vi "Generate Signal.vi"(8 "error in (no error)":errorcluster, 11 "Sampling Rate":dbl=10000000.0 format="%#_13p") -> (0 "error out":errorcluster, 2 "Waveform Out":waveform(cdb))   [LabVIEW 2018]
panel:
  out "Waveform Graph":dbl[](graph)
  out "Sampling Rate [Hz]":dbl
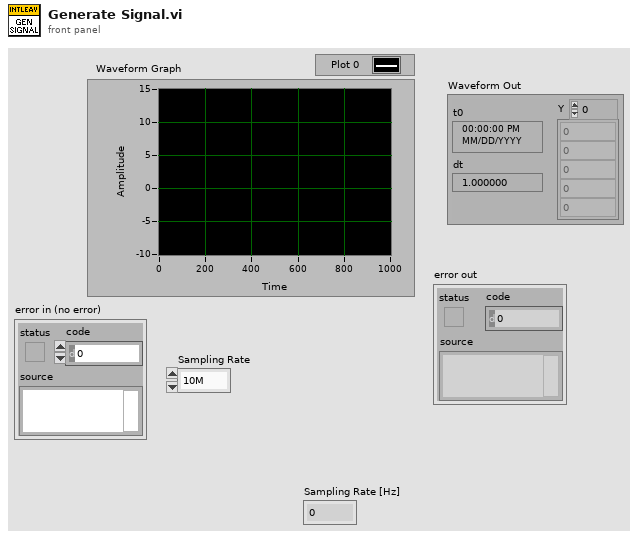
[diagram p1: front panel]
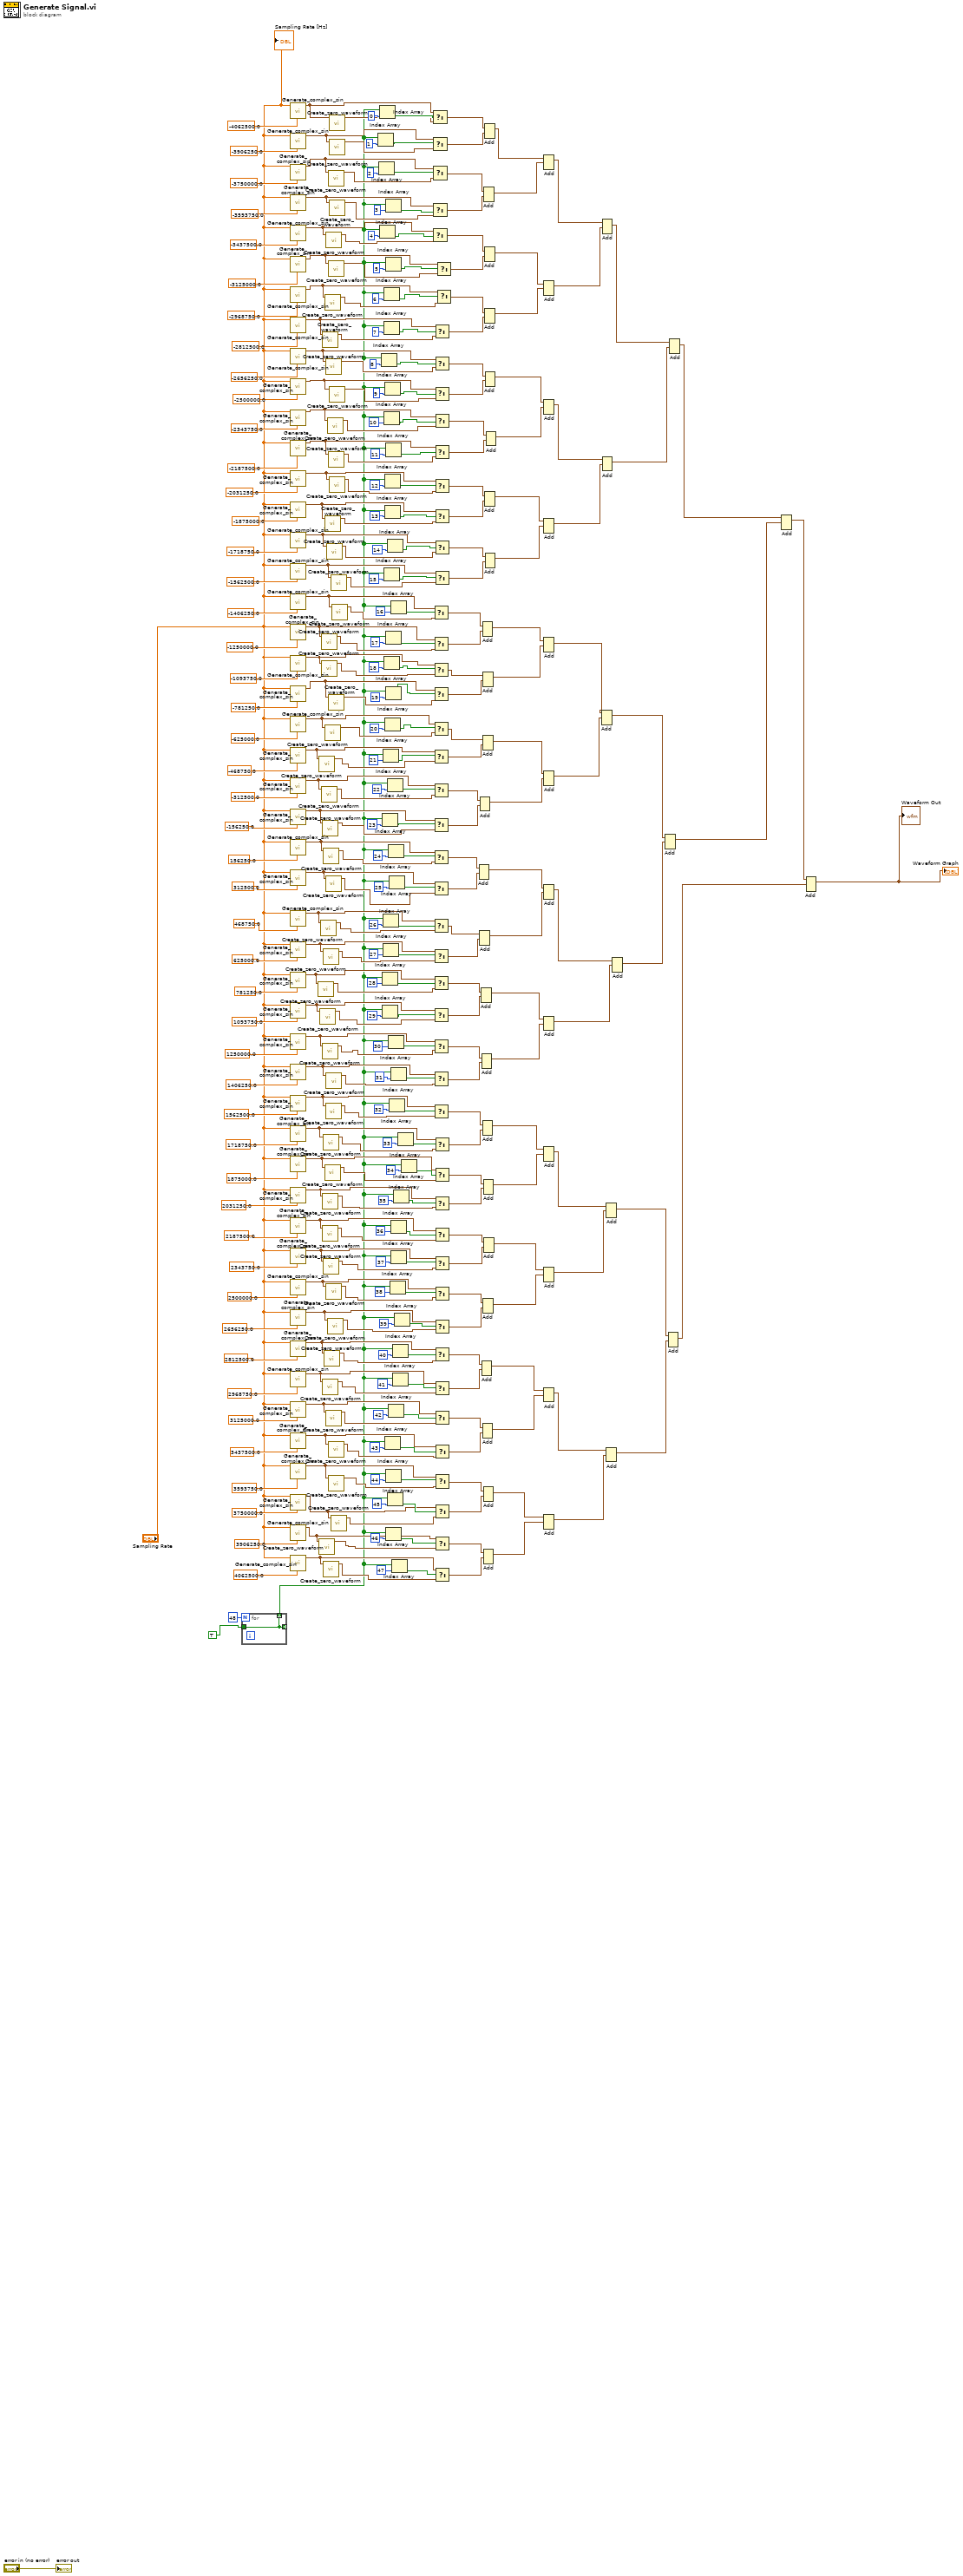
[diagram p0: block diagram]
diagram:
  n1 = for {
    N: 48 -> [_]
    tunnel: TRUE ("Boolean") -> [w341]
    tunnel: [w341] -> _ mode=indexing
    tunnel: [w341] -> w2 mode=indexing
  }
  n2 = call "Generate_complex_sin.vi"("Signal freq"=-4062500.0, "Sampling Rate [Hz]"="Sampling Rate") -> ("Waveform"=w102:waveform(cdb))  [unwired: 9 in]
  n3 = call "Generate_complex_sin.vi"("Signal freq"=-3906250.0, "Sampling Rate [Hz]"="Sampling Rate") -> ("Waveform"=w100:waveform(cdb))  [unwired: 9 in]
  n4 = call "Generate_complex_sin.vi"("Signal freq"=-3750000.0, "Sampling Rate [Hz]"="Sampling Rate") -> ("Waveform"=w97:waveform(cdb))  [unwired: 9 in]
  n5 = call "Generate_complex_sin.vi"("Signal freq"=-3593750.0, "Sampling Rate [Hz]"="Sampling Rate") -> ("Waveform"=w96:waveform(cdb))  [unwired: 9 in]
  n6 = call "Generate_complex_sin.vi"("Signal freq"=-3437500.0, "Sampling Rate [Hz]"="Sampling Rate") -> ("Waveform"=w93:waveform(cdb))  [unwired: 9 in]
  n7 = call "Generate_complex_sin.vi"("Signal freq"=-3125000.0, "Sampling Rate [Hz]"="Sampling Rate") -> ("Waveform"=w92:waveform(cdb))  [unwired: 9 in]
  n8 = call "Generate_complex_sin.vi"("Signal freq"=-2968750.0, "Sampling Rate [Hz]"="Sampling Rate") -> ("Waveform"=w89:waveform(cdb))  [unwired: 9 in]
  n9 = call "Generate_complex_sin.vi"("Signal freq"=-2812500.0, "Sampling Rate [Hz]"="Sampling Rate") -> ("Waveform"=w88:waveform(cdb))  [unwired: 9 in]
  n10 = call "Generate_complex_sin.vi"("Signal freq"=-2656250.0, "Sampling Rate [Hz]"="Sampling Rate") -> ("Waveform"=w86:waveform(cdb))  [unwired: 9 in]
  n11 = call "Generate_complex_sin.vi"("Signal freq"=-2500000.0, "Sampling Rate [Hz]"="Sampling Rate") -> ("Waveform"=w84:waveform(cdb))  [unwired: 9 in]
  n12 = call "Generate_complex_sin.vi"("Signal freq"=-2343750.0, "Sampling Rate [Hz]"="Sampling Rate") -> ("Waveform"=w82:waveform(cdb))  [unwired: 9 in]
  n13 = call "Generate_complex_sin.vi"("Signal freq"=-2187500.0, "Sampling Rate [Hz]"="Sampling Rate") -> ("Waveform"=w80:waveform(cdb))  [unwired: 9 in]
  n14 = call "Generate_complex_sin.vi"("Signal freq"=-2031250.0, "Sampling Rate [Hz]"="Sampling Rate") -> ("Waveform"=w78:waveform(cdb))  [unwired: 9 in]
  n15 = call "Generate_complex_sin.vi"("Signal freq"=-1875000.0, "Sampling Rate [Hz]"="Sampling Rate") -> ("Waveform"=w75:waveform(cdb))  [unwired: 9 in]
  n16 = call "Generate_complex_sin.vi"("Signal freq"=-1718750.0, "Sampling Rate [Hz]"="Sampling Rate") -> ("Waveform"=w74:waveform(cdb))  [unwired: 9 in]
  n17 = call "Generate_complex_sin.vi"("Signal freq"=-1562500.0, "Sampling Rate [Hz]"="Sampling Rate") -> ("Waveform"=w71:waveform(cdb))  [unwired: 9 in]
  n18 = call "Generate_complex_sin.vi"("Signal freq"=-1406250.0, "Sampling Rate [Hz]"="Sampling Rate") -> ("Waveform"=w69:waveform(cdb))  [unwired: 9 in]
  n19 = call "Generate_complex_sin.vi"("Signal freq"=-1250000.0, "Sampling Rate [Hz]"="Sampling Rate") -> ("Waveform"=w67:waveform(cdb))  [unwired: 9 in]
  n20 = call "Generate_complex_sin.vi"("Signal freq"=-1093750.0, "Sampling Rate [Hz]"="Sampling Rate") -> ("Waveform"=w65:waveform(cdb))  [unwired: 9 in]
  n21 = call "Generate_complex_sin.vi"("Signal freq"=-781250.0, "Sampling Rate [Hz]"="Sampling Rate") -> ("Waveform"=w63:waveform(cdb))  [unwired: 9 in]
  n22 = call "Generate_complex_sin.vi"("Signal freq"=-625000.0, "Sampling Rate [Hz]"="Sampling Rate") -> ("Waveform"=w61:waveform(cdb))  [unwired: 9 in]
  n23 = call "Generate_complex_sin.vi"("Signal freq"=-468750.0, "Sampling Rate [Hz]"="Sampling Rate") -> ("Waveform"=w59:waveform(cdb))  [unwired: 9 in]
  n24 = call "Generate_complex_sin.vi"("Signal freq"=-312500.0, "Sampling Rate [Hz]"="Sampling Rate") -> ("Waveform"=w57:waveform(cdb))  [unwired: 9 in]
  n25 = call "Generate_complex_sin.vi"("Signal freq"=-156250.0, "Sampling Rate [Hz]"="Sampling Rate") -> ("Waveform"=w55:waveform(cdb))  [unwired: 9 in]
  n26 = call "Generate_complex_sin.vi"("Signal freq"=156250.0, "Sampling Rate [Hz]"="Sampling Rate") -> ("Waveform"=w54:waveform(cdb))  [unwired: 9 in]
  n27 = call "Generate_complex_sin.vi"("Signal freq"=312500.0, "Sampling Rate [Hz]"="Sampling Rate") -> ("Waveform"=w51:waveform(cdb))  [unwired: 9 in]
  n28 = call "Generate_complex_sin.vi"("Signal freq"=468750.0, "Sampling Rate [Hz]"="Sampling Rate") -> ("Waveform"=w49:waveform(cdb))  [unwired: 9 in]
  n29 = call "Generate_complex_sin.vi"("Signal freq"=625000.0, "Sampling Rate [Hz]"="Sampling Rate") -> ("Waveform"=w47:waveform(cdb))  [unwired: 9 in]
  n30 = call "Generate_complex_sin.vi"("Signal freq"=781250.0, "Sampling Rate [Hz]"="Sampling Rate") -> ("Waveform"=w45:waveform(cdb))  [unwired: 9 in]
  n31 = call "Generate_complex_sin.vi"("Signal freq"=1093750.0, "Sampling Rate [Hz]"="Sampling Rate") -> ("Waveform"=w43:waveform(cdb))  [unwired: 9 in]
  n32 = call "Generate_complex_sin.vi"("Signal freq"=1250000.0, "Sampling Rate [Hz]"="Sampling Rate") -> ("Waveform"=w41:waveform(cdb))  [unwired: 9 in]
  n33 = call "Generate_complex_sin.vi"("Signal freq"=1406250.0, "Sampling Rate [Hz]"="Sampling Rate") -> ("Waveform"=w39:waveform(cdb))  [unwired: 9 in]
  n34 = call "Generate_complex_sin.vi"("Signal freq"=1562500.0, "Sampling Rate [Hz]"="Sampling Rate") -> ("Waveform"=w37:waveform(cdb))  [unwired: 9 in]
  n35 = call "Generate_complex_sin.vi"("Signal freq"=1718750.0, "Sampling Rate [Hz]"="Sampling Rate") -> ("Waveform"=w35:waveform(cdb))  [unwired: 9 in]
  n36 = call "Generate_complex_sin.vi"("Signal freq"=1875000.0, "Sampling Rate [Hz]"="Sampling Rate") -> ("Waveform"=w33:waveform(cdb))  [unwired: 9 in]
  n37 = call "Generate_complex_sin.vi"("Signal freq"=2031250.0, "Sampling Rate [Hz]"="Sampling Rate") -> ("Waveform"=w31:waveform(cdb))  [unwired: 9 in]
  n38 = call "Generate_complex_sin.vi"("Signal freq"=2187500.0, "Sampling Rate [Hz]"="Sampling Rate") -> ("Waveform"=w29:waveform(cdb))  [unwired: 9 in]
  n39 = call "Generate_complex_sin.vi"("Signal freq"=2343750.0, "Sampling Rate [Hz]"="Sampling Rate") -> ("Waveform"=w28:waveform(cdb))  [unwired: 9 in]
  n40 = call "Generate_complex_sin.vi"("Signal freq"=2500000.0, "Sampling Rate [Hz]"="Sampling Rate") -> ("Waveform"=w25:waveform(cdb))  [unwired: 9 in]
  n41 = call "Generate_complex_sin.vi"("Signal freq"=2656250.0, "Sampling Rate [Hz]"="Sampling Rate") -> ("Waveform"=w23:waveform(cdb))  [unwired: 9 in]
  n42 = call "Generate_complex_sin.vi"("Signal freq"=2812500.0, "Sampling Rate [Hz]"="Sampling Rate") -> ("Waveform"=w21:waveform(cdb))  [unwired: 9 in]
  n43 = call "Generate_complex_sin.vi"("Signal freq"=2968750.0, "Sampling Rate [Hz]"="Sampling Rate") -> ("Waveform"=w19:waveform(cdb))  [unwired: 9 in]
  n44 = call "Generate_complex_sin.vi"("Signal freq"=3125000.0, "Sampling Rate [Hz]"="Sampling Rate") -> ("Waveform"=w18:waveform(cdb))  [unwired: 9 in]
  n45 = call "Generate_complex_sin.vi"("Signal freq"=3437500.0, "Sampling Rate [Hz]"="Sampling Rate") -> ("Waveform"=w15:waveform(cdb))  [unwired: 9 in]
  n46 = call "Generate_complex_sin.vi"("Signal freq"=3593750.0, "Sampling Rate [Hz]"="Sampling Rate") -> ("Waveform"=w13:waveform(cdb))  [unwired: 9 in]
  n47 = call "Generate_complex_sin.vi"("Signal freq"=3750000.0, "Sampling Rate [Hz]"="Sampling Rate") -> ("Waveform"=w12:waveform(cdb))  [unwired: 9 in]
  n48 = call "Generate_complex_sin.vi"("Signal freq"=3906250.0, "Sampling Rate [Hz]"="Sampling Rate") -> ("Waveform"=w9:waveform(cdb))  [unwired: 9 in]
  n49 = call "Generate_complex_sin.vi"("Signal freq"=4062500.0, "Sampling Rate [Hz]"="Sampling Rate") -> ("Waveform"=w7:waveform(cdb))  [unwired: 9 in]
  n50 = call "Create_zero_waveform.vi"("Waveform in"=w45) -> ("Waveform out"=w46:waveform(cdb))  [unwired: 10 in]
  n51 = call "Create_zero_waveform.vi"("Waveform in"=w59) -> ("Waveform out"=w60:waveform(cdb))  [unwired: 10 in]
  n52 = call "Create_zero_waveform.vi"("Waveform in"=w9) -> ("Waveform out"=w10:waveform(cdb))  [unwired: 10 in]
  n53 = call "Create_zero_waveform.vi"("Waveform in"=w43) -> ("Waveform out"=w44:waveform(cdb))  [unwired: 10 in]
  n54 = call "Create_zero_waveform.vi"("Waveform in"=w49) -> ("Waveform out"=w50:waveform(cdb))  [unwired: 10 in]
  n55 = call "Create_zero_waveform.vi"("Waveform in"=w67) -> ("Waveform out"=w68:waveform(cdb))  [unwired: 10 in]
  n56 = call "Create_zero_waveform.vi"("Waveform in"=w65) -> ("Waveform out"=w66:waveform(cdb))  [unwired: 10 in]
  n57 = call "Create_zero_waveform.vi"("Waveform in"=w57) -> ("Waveform out"=w58:waveform(cdb))  [unwired: 10 in]
  n58 = call "Create_zero_waveform.vi"("Waveform in"=w88) -> ("Waveform out"=w87:waveform(cdb))  [unwired: 10 in]
  n59 = call "Create_zero_waveform.vi"("Waveform in"=w41) -> ("Waveform out"=w42:waveform(cdb))  [unwired: 10 in]
  n60 = call "Create_zero_waveform.vi"("Waveform in"=w29) -> ("Waveform out"=w30:waveform(cdb))  [unwired: 10 in]
  n61 = call "Create_zero_waveform.vi"("Waveform in"=w55) -> ("Waveform out"=w56:waveform(cdb))  [unwired: 10 in]
  n62 = call "Create_zero_waveform.vi"("Waveform in"=w31) -> ("Waveform out"=w32:waveform(cdb))  [unwired: 10 in]
  n63 = call "Create_zero_waveform.vi"("Waveform in"=w19) -> ("Waveform out"=w20:waveform(cdb))  [unwired: 10 in]
  n64 = call "Create_zero_waveform.vi"("Waveform in"=w47) -> ("Waveform out"=w48:waveform(cdb))  [unwired: 10 in]
  n65 = call "Create_zero_waveform.vi"("Waveform in"=w35) -> ("Waveform out"=w36:waveform(cdb))  [unwired: 10 in]
  n66 = call "Create_zero_waveform.vi"("Waveform in"=w28) -> ("Waveform out"=w27:waveform(cdb))  [unwired: 10 in]
  n67 = call "Create_zero_waveform.vi"("Waveform in"=w7) -> ("Waveform out"=w8:waveform(cdb))  [unwired: 10 in]
  n68 = call "Create_zero_waveform.vi"("Waveform in"=w54) -> ("Waveform out"=w53:waveform(cdb))  [unwired: 10 in]
  n69 = call "Create_zero_waveform.vi"("Waveform in"=w21) -> ("Waveform out"=w22:waveform(cdb))  [unwired: 10 in]
  n70 = call "Create_zero_waveform.vi"("Waveform in"=w33) -> ("Waveform out"=w34:waveform(cdb))  [unwired: 10 in]
  n71 = call "Create_zero_waveform.vi"("Waveform in"=w89) -> ("Waveform out"=w90:waveform(cdb))  [unwired: 10 in]
  n72 = call "Create_zero_waveform.vi"("Waveform in"=w75) -> ("Waveform out"=w76:waveform(cdb))  [unwired: 10 in]
  n73 = call "Create_zero_waveform.vi"("Waveform in"=w61) -> ("Waveform out"=w62:waveform(cdb))  [unwired: 10 in]
  n74 = call "Create_zero_waveform.vi"("Waveform in"=w86) -> ("Waveform out"=w85:waveform(cdb))  [unwired: 10 in]
  n75 = call "Create_zero_waveform.vi"("Waveform in"=w51) -> ("Waveform out"=w52:waveform(cdb))  [unwired: 10 in]
  n76 = call "Create_zero_waveform.vi"("Waveform in"=w37) -> ("Waveform out"=w38:waveform(cdb))  [unwired: 10 in]
  n77 = call "Create_zero_waveform.vi"("Waveform in"=w18) -> ("Waveform out"=w17:waveform(cdb))  [unwired: 10 in]
  n78 = call "Create_zero_waveform.vi"("Waveform in"=w93) -> ("Waveform out"=w94:waveform(cdb))  [unwired: 10 in]
  n79 = call "Create_zero_waveform.vi"("Waveform in"=w39) -> ("Waveform out"=w40:waveform(cdb))  [unwired: 10 in]
  n80 = call "Create_zero_waveform.vi"("Waveform in"=w25) -> ("Waveform out"=w26:waveform(cdb))  [unwired: 10 in]
  n81 = call "Create_zero_waveform.vi"("Waveform in"=w74) -> ("Waveform out"=w73:waveform(cdb))  [unwired: 10 in]
  n82 = call "Create_zero_waveform.vi"("Waveform in"=w82) -> ("Waveform out"=w81:waveform(cdb))  [unwired: 10 in]
  n83 = call "Create_zero_waveform.vi"("Waveform in"=w23) -> ("Waveform out"=w24:waveform(cdb))  [unwired: 10 in]
  n84 = call "Create_zero_waveform.vi"("Waveform in"=w97) -> ("Waveform out"=w98:waveform(cdb))  [unwired: 10 in]
  n85 = call "Create_zero_waveform.vi"("Waveform in"=w15) -> ("Waveform out"=w16:waveform(cdb))  [unwired: 10 in]
  n86 = call "Create_zero_waveform.vi"("Waveform in"=w92) -> ("Waveform out"=w91:waveform(cdb))  [unwired: 10 in]
  n87 = call "Create_zero_waveform.vi"("Waveform in"=w80) -> ("Waveform out"=w79:waveform(cdb))  [unwired: 10 in]
  n88 = call "Create_zero_waveform.vi"("Waveform in"=w63) -> ("Waveform out"=w64:waveform(cdb))  [unwired: 10 in]
  n89 = call "Create_zero_waveform.vi"("Waveform in"=w13) -> ("Waveform out"=w14:waveform(cdb))  [unwired: 10 in]
  n90 = call "Create_zero_waveform.vi"("Waveform in"=w78) -> ("Waveform out"=w77:waveform(cdb))  [unwired: 10 in]
  n91 = call "Create_zero_waveform.vi"("Waveform in"=w102) -> ("Waveform out"=w101:waveform(cdb))  [unwired: 10 in]
  n92 = call "Create_zero_waveform.vi"("Waveform in"=w100) -> ("Waveform out"=w99:waveform(cdb))  [unwired: 10 in]
  n93 = call "Create_zero_waveform.vi"("Waveform in"=w96) -> ("Waveform out"=w95:waveform(cdb))  [unwired: 10 in]
  n94 = call "Create_zero_waveform.vi"("Waveform in"=w84) -> ("Waveform out"=w83:waveform(cdb))  [unwired: 10 in]
  n95 = call "Create_zero_waveform.vi"("Waveform in"=w12) -> ("Waveform out"=w11:waveform(cdb))  [unwired: 10 in]
  n96 = call "Create_zero_waveform.vi"("Waveform in"=w71) -> ("Waveform out"=w72:waveform(cdb))  [unwired: 10 in]
  n97 = call "Create_zero_waveform.vi"("Waveform in"=w69) -> ("Waveform out"=w70:waveform(cdb))  [unwired: 10 in]
  n98 = Index Array(array=w2, index=1) -> (element=w242:bool)
  n99 = Index Array(array=w2, index=2) -> (element=w241:bool)
  n100 = Index Array(array=w2, index=0) -> (element=w243:bool)
  n101 = Index Array(array=w2, index=4) -> (element=w239:bool)
  n102 = Index Array(array=w2, index=8) -> (element=w235:bool)
  n103 = Index Array(array=w2, index=23) -> (element=w220:bool)
  n104 = Index Array(array=w2, index=28) -> (element=w215:bool)
  n105 = Index Array(array=w2, index=29) -> (element=w214:bool)
  n106 = Index Array(array=w2, index=21) -> (element=w222:bool)
  n107 = Index Array(array=w2, index=26) -> (element=w217:bool)
  n108 = Index Array(array=w2, index=27) -> (element=w216:bool)
  n109 = Index Array(array=w2, index=6) -> (element=w237:bool)
  n110 = Index Array(array=w2, index=7) -> (element=w236:bool)
  n111 = Index Array(array=w2, index=10) -> (element=w233:bool)
  n112 = Index Array(array=w2, index=15) -> (element=w228:bool)
  n113 = Index Array(array=w2, index=18) -> (element=w225:bool)
  n114 = Index Array(array=w2, index=20) -> (element=w223:bool)
  n115 = Index Array(array=w2, index=9) -> (element=w234:bool)
  n116 = Index Array(array=w2, index=12) -> (element=w231:bool)
  n117 = Index Array(array=w2, index=13) -> (element=w230:bool)
  n118 = Index Array(array=w2, index=43) -> (element=w200:bool)
  n119 = Index Array(array=w2, index=5) -> (element=w238:bool)
  n120 = Index Array(array=w2, index=11) -> (element=w232:bool)
  n121 = Index Array(array=w2, index=17) -> (element=w226:bool)
  n122 = Index Array(array=w2, index=19) -> (element=w224:bool)
  n123 = Index Array(array=w2, index=44) -> (element=w199:bool)
  n124 = Index Array(array=w2, index=46) -> (element=w197:bool)
  n125 = Index Array(array=w2, index=3) -> (element=w240:bool)
  n126 = Index Array(array=w2, index=22) -> (element=w221:bool)
  n127 = Index Array(array=w2, index=45) -> (element=w198:bool)
  n128 = Index Array(array=w2, index=14) -> (element=w229:bool)
  n129 = Index Array(array=w2, index=24) -> (element=w219:bool)
  n130 = Index Array(array=w2, index=30) -> (element=w213:bool)
  n131 = Index Array(array=w2, index=42) -> (element=w201:bool)
  n132 = Index Array(array=w2, index=25) -> (element=w218:bool)
  n133 = Index Array(array=w2, index=32) -> (element=w211:bool)
  n134 = Index Array(array=w2, index=38) -> (element=w205:bool)
  n135 = Index Array(array=w2, index=16) -> (element=w227:bool)
  n136 = Index Array(array=w2, index=36) -> (element=w207:bool)
  n137 = Index Array(array=w2, index=31) -> (element=w212:bool)
  n138 = Index Array(array=w2, index=37) -> (element=w206:bool)
  n139 = Index Array(array=w2, index=47) -> (element=w196:bool)
  n140 = Index Array(array=w2, index=41) -> (element=w202:bool)
  n141 = Index Array(array=w2, index=40) -> (element=w203:bool)
  n142 = Index Array(array=w2, index=35) -> (element=w208:bool)
  n143 = Index Array(array=w2, index=39) -> (element=w204:bool)
  n144 = Index Array(array=w2, index=33) -> (element=w210:bool)
  n145 = Index Array(array=w2, index=34) -> (element=w209:bool)
  n146 = Select(t=w102, s=w243, f=w101) -> (s? t:f=w195:waveform(cdb))
  n147 = Select(t=w100, s=w242, f=w99) -> (s? t:f=w194:waveform(cdb))
  n148 = Select(t=w97, s=w241, f=w98) -> (s? t:f=w193:waveform(cdb))
  n149 = Select(t=w96, s=w240, f=w95) -> (s? t:f=w192:waveform(cdb))
  n150 = Select(t=w93, s=w239, f=w94) -> (s? t:f=w190:waveform(cdb))
  n151 = Select(t=w69, s=w227, f=w70) -> (s? t:f=w179:waveform(cdb))
  n152 = Select(t=w67, s=w226, f=w68) -> (s? t:f=w178:waveform(cdb))
  n153 = Select(t=w65, s=w225, f=w66) -> (s? t:f=w177:waveform(cdb))
  n154 = Select(t=w63, s=w224, f=w64) -> (s? t:f=w176:waveform(cdb))
  n155 = Select(t=w61, s=w223, f=w62) -> (s? t:f=w175:waveform(cdb))
  n156 = Select(t=w59, s=w222, f=w60) -> (s? t:f=w174:waveform(cdb))
  n157 = Select(t=w57, s=w221, f=w58) -> (s? t:f=w173:waveform(cdb))
  n158 = Select(t=w55, s=w220, f=w56) -> (s? t:f=w172:waveform(cdb))
  n159 = Select(t=w54, s=w219, f=w53) -> (s? t:f=w170:waveform(cdb))
  n160 = Select(t=w51, s=w218, f=w52) -> (s? t:f=w171:waveform(cdb))
  n161 = Select(t=w49, s=w217, f=w50) -> (s? t:f=w169:waveform(cdb))
  n162 = Select(t=w47, s=w216, f=w48) -> (s? t:f=w168:waveform(cdb))
  n163 = Select(t=w45, s=w215, f=w46) -> (s? t:f=w166:waveform(cdb))
  n164 = Select(t=w43, s=w214, f=w44) -> (s? t:f=w167:waveform(cdb))
  n165 = Select(t=w41, s=w213, f=w42) -> (s? t:f=w164:waveform(cdb))
  n166 = Select(t=w39, s=w212, f=w40) -> (s? t:f=w165:waveform(cdb))
  n167 = Select(t=w37, s=w211, f=w38) -> (s? t:f=w162:waveform(cdb))
  n168 = Select(t=w88, s=w236, f=w87) -> (s? t:f=w188:waveform(cdb))
  n169 = Select(t=w86, s=w235, f=w85) -> (s? t:f=w187:waveform(cdb))
  n170 = Select(t=w84, s=w234, f=w83) -> (s? t:f=w186:waveform(cdb))
  n171 = Select(t=w82, s=w233, f=w81) -> (s? t:f=w185:waveform(cdb))
  n172 = Select(t=w80, s=w232, f=w79) -> (s? t:f=w184:waveform(cdb))
  n173 = Select(t=w78, s=w231, f=w77) -> (s? t:f=w183:waveform(cdb))
  n174 = Select(t=w75, s=w230, f=w76) -> (s? t:f=w182:waveform(cdb))
  n175 = Select(t=w74, s=w229, f=w73) -> (s? t:f=w181:waveform(cdb))
  n176 = Select(t=w71, s=w228, f=w72) -> (s? t:f=w180:waveform(cdb))
  n177 = Select(t=w35, s=w210, f=w36) -> (s? t:f=w163:waveform(cdb))
  n178 = Select(t=w33, s=w209, f=w34) -> (s? t:f=w160:waveform(cdb))
  n179 = Select(t=w31, s=w208, f=w32) -> (s? t:f=w161:waveform(cdb))
  n180 = Select(t=w29, s=w207, f=w30) -> (s? t:f=w158:waveform(cdb))
  n181 = Select(t=w28, s=w206, f=w27) -> (s? t:f=w159:waveform(cdb))
  n182 = Select(t=w25, s=w205, f=w26) -> (s? t:f=w156:waveform(cdb))
  n183 = Select(t=w23, s=w204, f=w24) -> (s? t:f=w157:waveform(cdb))
  n184 = Select(t=w21, s=w203, f=w22) -> (s? t:f=w154:waveform(cdb))
  n185 = Select(t=w19, s=w202, f=w20) -> (s? t:f=w155:waveform(cdb))
  n186 = Select(t=w18, s=w201, f=w17) -> (s? t:f=w153:waveform(cdb))
  n187 = Select(t=w15, s=w200, f=w16) -> (s? t:f=w152:waveform(cdb))
  n188 = Select(t=w13, s=w199, f=w14) -> (s? t:f=w151:waveform(cdb))
  n189 = Select(t=w12, s=w198, f=w11) -> (s? t:f=w150:waveform(cdb))
  n190 = Select(t=w9, s=w197, f=w10) -> (s? t:f=w149:waveform(cdb))
  n191 = Select(t=w7, s=w196, f=w8) -> (s? t:f=w148:waveform(cdb))
  n192 = Select(t=w92, s=w238, f=w91) -> (s? t:f=w191:waveform(cdb))
  n193 = Select(t=w89, s=w237, f=w90) -> (s? t:f=w189:waveform(cdb))
  n194 = Add(1:w171, 2:w170) -> (0:w134:waveform(cdb))  [unwired: 1 in, 1 out]
  n195 = Add(1:w168, 2:w169) -> (0:w135:waveform(cdb))  [unwired: 1 in, 1 out]
  n196 = Add(1:w172, 2:w173) -> (0:w137:waveform(cdb))  [unwired: 1 in, 1 out]
  n197 = Add(1:w167, 2:w166) -> (0:w132:waveform(cdb))  [unwired: 1 in, 1 out]
  n198 = Add(1:w165, 2:w164) -> (0:w133:waveform(cdb))  [unwired: 1 in, 1 out]
  n199 = Add(1:w155, 2:w154) -> (0:w126:waveform(cdb))  [unwired: 1 in, 1 out]
  n200 = Add(1:w178, 2:w179) -> (0:w138:waveform(cdb))  [unwired: 1 in, 1 out]
  n201 = Add(1:w163, 2:w162) -> (0:w130:waveform(cdb))  [unwired: 1 in, 1 out]
  n202 = Add(1:w152, 2:w153) -> (0:w127:waveform(cdb))  [unwired: 1 in, 1 out]
  n203 = Add(1:w176, 2:w177) -> (0:w139:waveform(cdb))  [unwired: 1 in, 1 out]
  n204 = Add(1:w174, 2:w175) -> (0:w136:waveform(cdb))  [unwired: 1 in, 1 out]
  n205 = Add(1:w157, 2:w156) -> (0:w129:waveform(cdb))  [unwired: 1 in, 1 out]
  n206 = Add(1:w161, 2:w160) -> (0:w131:waveform(cdb))  [unwired: 1 in, 1 out]
  n207 = Add(1:w150, 2:w151) -> (0:w124:waveform(cdb))  [unwired: 1 in, 1 out]
  n208 = Add(1:w148, 2:w149) -> (0:w125:waveform(cdb))  [unwired: 1 in, 1 out]
  n209 = Add(1:w192, 2:w193) -> (0:w146:waveform(cdb))  [unwired: 1 in, 1 out]
  n210 = Add(1:w159, 2:w158) -> (0:w128:waveform(cdb))  [unwired: 1 in, 1 out]
  n211 = Add(1:w194, 2:w195) -> (0:w147:waveform(cdb))  [unwired: 1 in, 1 out]
  n212 = Add(1:w191, 2:w190) -> (0:w144:waveform(cdb))  [unwired: 1 in, 1 out]
  n213 = Add(1:w188, 2:w189) -> (0:w145:waveform(cdb))  [unwired: 1 in, 1 out]
  n214 = Add(1:w182, 2:w183) -> (0:w140:waveform(cdb))  [unwired: 1 in, 1 out]
  n215 = Add(1:w186, 2:w187) -> (0:w142:waveform(cdb))  [unwired: 1 in, 1 out]
  n216 = Add(1:w180, 2:w181) -> (0:w141:waveform(cdb))  [unwired: 1 in, 1 out]
  n217 = Add(1:w184, 2:w185) -> (0:w143:waveform(cdb))  [unwired: 1 in, 1 out]
  n218 = Add(1:w146, 2:w147) -> (0:w6:waveform(cdb))  [unwired: 1 in, 1 out]
  n219 = Add(1:w145, 2:w144) -> (0:w123:waveform(cdb))  [unwired: 1 in, 1 out]
  n220 = Add(1:w143, 2:w142) -> (0:w122:waveform(cdb))  [unwired: 1 in, 1 out]
  n221 = Add(1:w141, 2:w140) -> (0:w121:waveform(cdb))  [unwired: 1 in, 1 out]
  n222 = Add(1:w139, 2:w138) -> (0:w120:waveform(cdb))  [unwired: 1 in, 1 out]
  n223 = Add(1:w137, 2:w136) -> (0:w119:waveform(cdb))  [unwired: 1 in, 1 out]
  n224 = Add(1:w135, 2:w134) -> (0:w118:waveform(cdb))  [unwired: 1 in, 1 out]
  n225 = Add(1:w133, 2:w132) -> (0:w117:waveform(cdb))  [unwired: 1 in, 1 out]
  n226 = Add(1:w131, 2:w130) -> (0:w116:waveform(cdb))  [unwired: 1 in, 1 out]
  n227 = Add(1:w129, 2:w128) -> (0:w115:waveform(cdb))  [unwired: 1 in, 1 out]
  n228 = Add(1:w127, 2:w126) -> (0:w114:waveform(cdb))  [unwired: 1 in, 1 out]
  n229 = Add(1:w125, 2:w124) -> (0:w113:waveform(cdb))  [unwired: 1 in, 1 out]
  n230 = Add(1:w119, 2:w120) -> (0:w109:waveform(cdb))  [unwired: 1 in, 1 out]
  n231 = Add(1:w123, 2:w6) -> (0:w112:waveform(cdb))  [unwired: 1 in, 1 out]
  n232 = Add(1:w121, 2:w122) -> (0:w111:waveform(cdb))  [unwired: 1 in, 1 out]
  n233 = Add(1:w115, 2:w116) -> (0:w107:waveform(cdb))  [unwired: 1 in, 1 out]
  n234 = Add(1:w113, 2:w114) -> (0:w108:waveform(cdb))  [unwired: 1 in, 1 out]
  n235 = Add(1:w117, 2:w118) -> (0:w110:waveform(cdb))  [unwired: 1 in, 1 out]
  n236 = Add(1:w110, 2:w109) -> (0:w105:waveform(cdb))  [unwired: 1 in, 1 out]
  n237 = Add(1:w108, 2:w107) -> (0:w104:waveform(cdb))  [unwired: 1 in, 1 out]
  n238 = Add(1:w111, 2:w112) -> (0:w106:waveform(cdb))  [unwired: 1 in, 1 out]
  n239 = Add(1:w105, 2:w106) -> (0:w103:waveform(cdb))  [unwired: 1 in, 1 out]
  n240 = Add(1:w104, 2:w103) -> (0:→"Waveform Out" →"Waveform Graph":waveform(cdb))  [unwired: 1 in, 1 out]
  "error out" <- "error in (no error)"
  "Sampling Rate [Hz]" <- "Sampling Rate"
